vi "Test Create Multiple Reports.vi"(8 "error in (no error)":errorcluster, 11 "XML Report Test in":refnum<class "XML Report Test.lvclass">) -> (0 "error out":errorcluster, 3 "XML Report Test out":refnum<class "XML Report Test.lvclass">)   [LabVIEW 2020, in "XML Report Test.lvclass"]
uses:
  XML Report Test.lvclass
  XML Report Test.lvclass/XML Report Test.ctl
  source/Plugins/XML Report/XML Report.lvclass
  <vilib>/Astemes/LUnit/Test Case.lvclass
  C:/Program Files (x86)/National Instruments/LabVIEW 2020/vi.lib/Astemes/LUnit/Test Case.lvclass
  C:/Program Files (x86)/National Instruments/LabVIEW 2020/vi.lib/Astemes/LUnit/LUnit Runnable.lvclass
  C:/git/astemes-lunit/tests/XML Report Test/XML Report Test.lvclass
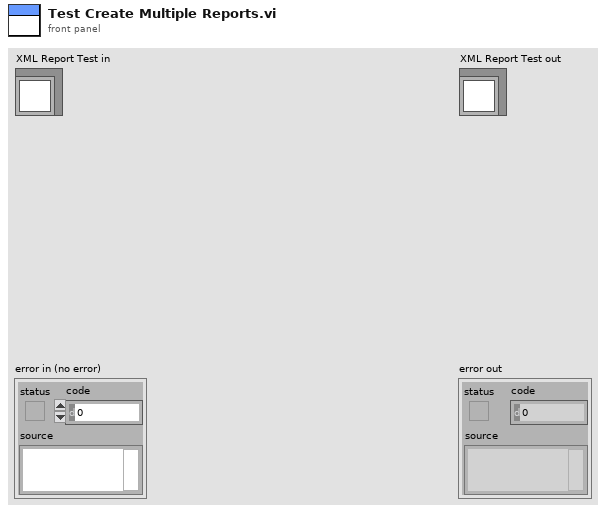
[diagram p1: front panel]
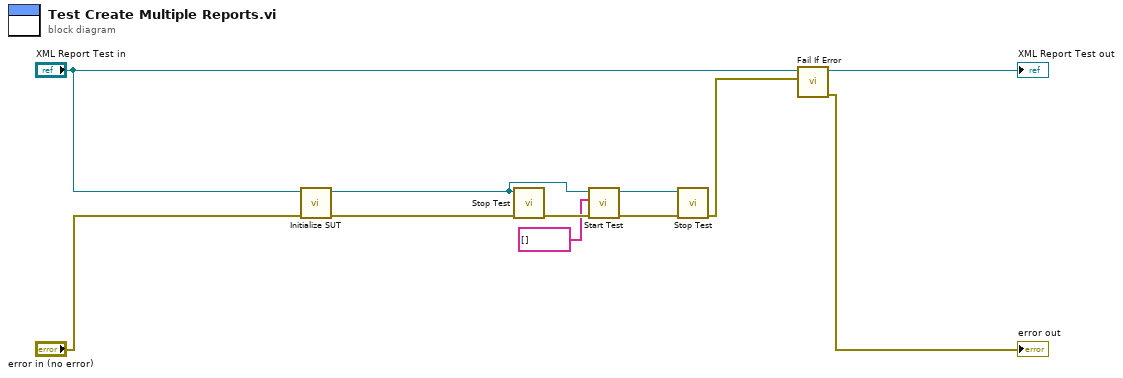
[diagram p0: block diagram]
diagram:
  n1 = call "Initialize SUT.vi"("error in (no error)"="error in (no error)", "XML Report Test in"="XML Report Test in") -> ("error out"=w3:errorcluster, "XML Report out"=w2:refnum<class "XML Report.lvclass">)  [unwired: 8 in]
  n2 = call-dynamic "Stop Test.vi"("error in (no error)"=w3, "XML Report In"=w2) -> ("error out"=w5:errorcluster)  [unwired: 8 in, 1 out]
  n3 = call-dynamic "Start Test.vi"("error in (no error)"=w5, "Tests"=string[] [], "XML Report In"=w2) -> ("error out"=w6:errorcluster, "XML Report Out"=w7:refnum<class "XML Report.lvclass">)  [unwired: 7 in]
  n4 = call-dynamic "Stop Test.vi"("error in (no error)"=w6, "XML Report In"=w7) -> ("error out"=w4:errorcluster)  [unwired: 8 in, 1 out]
  n5 = call <vilib>:"Fail If Error.vi"("Assert error"=w4, "LUnit Test Case In"="XML Report Test in") -> ("error out"=→"error out":errorcluster, "LUnit Test Case Out"=→"XML Report Test out":refnum<class "XML Report Test.lvclass">)  [unwired: 8 in]
